vi "Perform Action.vi"(8 "error in":errorcluster, 9 "Input":variant, 10 "Point Ident":string, 11 "MSS Target Actor in":refnum<class "MSS Target Actor.lvclass">) -> (0 "error out":errorcluster, 1 "Output":variant, 3 "MSS Target Actor out":refnum<class "MSS Target Actor.lvclass">)   [LabVIEW 2023, in "MSS Target Actor.lvlib" / "MSS Target Actor.lvclass"]
uses:
  MSS Target Actor.lvclass
  MSS Target Actor.lvclass/MSS Target Actor.ctl
  Measure and Stimulus Subsystems/Measure and Stimulus Subsystems.lvclass
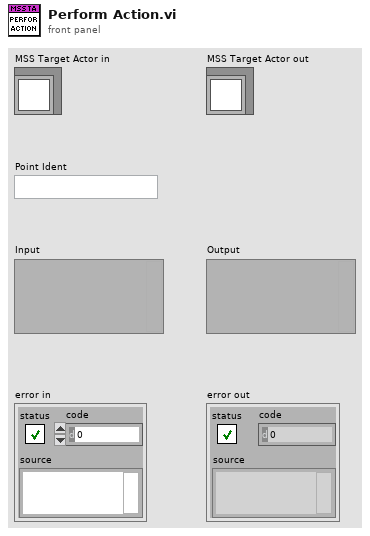
[diagram p1: front panel]
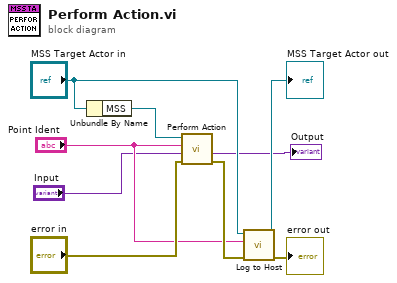
[diagram p0: block diagram]
diagram:
  n1 = Unbundle By Name("MSS Target Actor in") -> ("MSS"=w9:refnum<class "Measure and Stimulus Subsystems.lvclass">)
  n2 = call "Perform Action.vi"("error in"="error in", "Input"="Input", "Point Ident"="Point Ident", "MSS in"=w9) -> ("error out"=w7:errorcluster, "Output"=→"Output":variant)  [unwired: 4 in, 2 out]
  n3 = call "Log to Host.vi"("error in"=w7, "Detail"="Point Ident", "MSS Target Actor in"="MSS Target Actor in") -> ("error out"=→"error out":errorcluster, "MSS Target Actor out"=→"MSS Target Actor out":refnum<class "MSS Target Actor.lvclass">)  [unwired: 7 in]
